vi "Get Waveform Sweep Status.vi"(8 "error in (no error)":errorcluster, 10 "index":i32, 11 "Waveforms in":waveform(dbl)[](array[waveform])) -> (0 "error out":errorcluster, 2 "sweep status":T1, 3 "Waveforms out":waveform(dbl)[](array[waveform]))   [LabVIEW 2019, in "Generator.lvclass"]
uses:
  Generator.lvclass
  typedefs/Generator.Sweep Status--enum.ctl
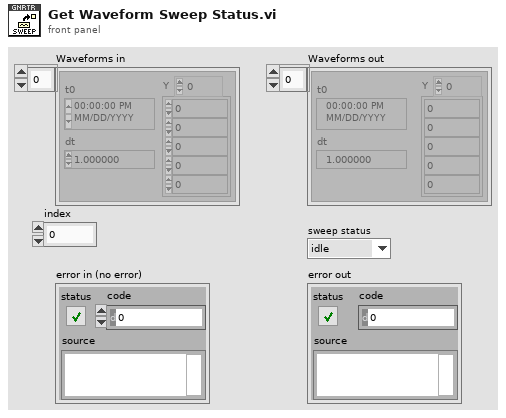
[diagram p1: front panel]
types:
  T1 = typedef "Generator.lvclass/Generator.Sweep Status--enum.ctl" = enum16{"idle", "initializing", "waiting", "sweeping", "stopping"}
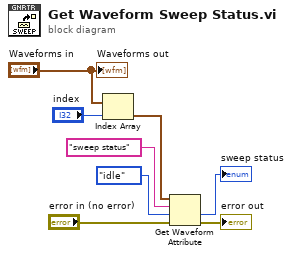
[diagram p0: block diagram]
diagram:
  n1 = Index Array(array="Waveforms in", index="index") -> (element=w7:waveform(dbl))
  n2 = Get Waveform Attribute(4:"error in (no error)", 5:Generator.Sweep_Status--enum."idle" ("sweep status"), 6:"sweep status" ("name"), 7:w7) -> (0:→"error out":errorcluster, 1:→"sweep status":T1)  [unwired: 2 out]
  "Waveforms out" <- "Waveforms in"
